vi "Get Service Address.vi"(8 "error in":errorcluster, 11 "service to run":string="GetSineSignal_LabVIEW") -> (0 "error out":errorcluster, 3 "service address":string)   [LabVIEW 2020, in "Client.lvlib"]
uses:
  <vilib>/MeasurementLink/MeasurementLink Discovery Client/RPC Messages/ni_measurementlink_discovery_v1_ResolveServiceRequest.ctl
  <vilib>/MeasurementLink/MeasurementLink Discovery Client/RPC Messages/ni_measurementlink_discovery_v1_EnumerateServicesRequest.ctl
  Client.lvlib
  <vilib>/MeasurementLink/MeasurementLink Discovery Client/MeasurementLink Discovery Client.lvlib
  <vilib>/MeasurementLink/MeasurementLink Discovery V1/MeasurementLink Discovery V1.lvlib
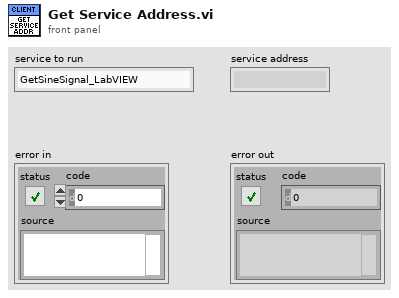
[diagram p1: front panel]
types:
  T1 = typedef "MeasurementLink Discovery Client.lvlib/ni_measurementlink_discovery_v1_EnumerateServicesRequest.ctl" = cluster{"provided_interface":string}
  T2 = typedef "MeasurementLink Discovery Client.lvlib/ni_measurementlink_discovery_v1_ResolveServiceRequest.ctl" = cluster{"provided_interface":string, "service_class":string}
  T3 = typedef "grpc-lvsupport-release.lvlib/grpcId.ctl" = u64
  T4 = typedef "MeasurementLink Discovery Client.lvlib/ni_measurementlink_discovery_v1_ServiceLocation.ctl" = cluster{"location":string, "insecure_port":string, "ssl_authenticated_port":string}
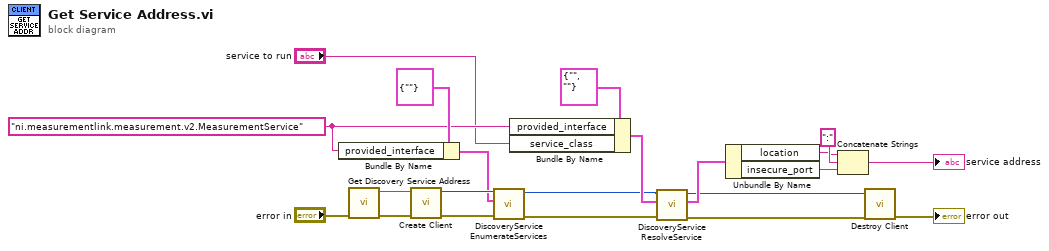
[diagram p0: block diagram]
diagram:
  w2 = "ni.measurementlink.measurement.v2.MeasurementService" ("provided_interface")
  n1 = Bundle By Name(cluster=T1 {"provided_interface"=""} ("Request Data"), "provided_interface"=w2) -> (w3:T1)
  n2 = call <vilib>:"Get Discovery Service Address.vi"("error in"="error in") -> ("error out"=w7:errorcluster, "address"=w6:string)  [unwired: 9 in]
  n3 = call <vilib>:"Create Client.vi"("error in"=w7, "address"=w6) -> ("error out"=w9:errorcluster, "gRPC ID Out"=w8:T3)  [unwired: 8 in]
  n4 = call <vilib>:"DiscoveryService EnumerateServices.vi"("error in"=w9, "Request Data"=w3, "gRPC ID"=w8) -> ("error out"=w11:errorcluster, "gRPC ID out"=w10:T3)  [unwired: 6 in, 1 out]
  n5 = Bundle By Name(cluster=T2 {"provided_interface"="", "service_class"=""} ("Request Data"), "provided_interface"=w2, "service_class"="service to run") -> (w15:T2)
  n6 = call <vilib>:"DiscoveryService ResolveService.vi"("error in"=w11, "Request Data"=w15, "gRPC ID"=w10) -> ("error out"=w12:errorcluster, "Response Data"=w16:T4, "gRPC ID out"=w13:T3)  [unwired: 6 in]
  n7 = Unbundle By Name(w16) -> ("location"=w17:string, "insecure_port"=w19:string)
  n8 = Concatenate Strings(w17, ":" ("string"), w19) -> (→"service address":string)
  n9 = call <vilib>:"Destroy Client.vi"("error in"=w12, "gRPC ID"=w13) -> ("error out"=→"error out":errorcluster)  [unwired: 9 in]
